vi "Write NmdNumericSize.vi"(5 "NmdNumericSize":T1, 9 "NamedNumeric in":refnum<class "NamedNumeric.lvclass">) -> (3 "NamedNumeric out":refnum<class "NamedNumeric.lvclass">)   [LabVIEW 2014, in "NamedNumeric.lvclass"]
uses:
  NamedNumeric.lvclass
  <vilib>/Utility/miscctls.llb/LVBoundsTypeDef.ctl
  NamedNumeric.lvclass/NamedNumeric.ctl
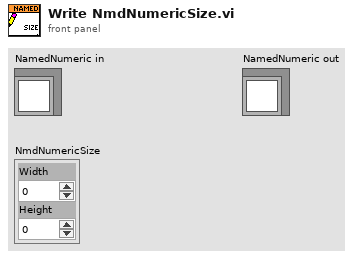
[diagram p1: front panel]
types:
  T1 = typedef "LVBoundsTypeDef.ctl" = cluster{"Width":u32, "Height":u32}
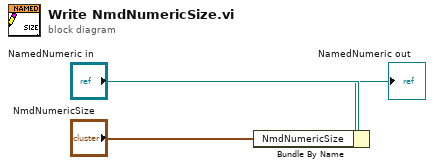
[diagram p0: block diagram]
diagram:
  n1 = Bundle By Name(cluster="NamedNumeric in", "NmdNumericSize"="NmdNumericSize") -> (→"NamedNumeric out":refnum<class "NamedNumeric.lvclass">)
